vi "VI-Get KObject Descendants.vi"(11 "error in (no error)":errorcluster) -> (4 "KObject descendants":string[](array[string]), 15 "error out":errorcluster)   [LabVIEW 2015]
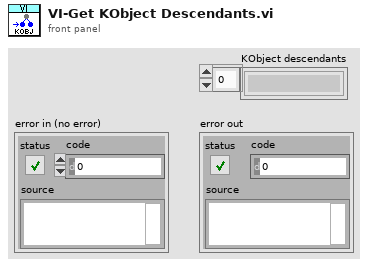
[diagram p1: front panel]
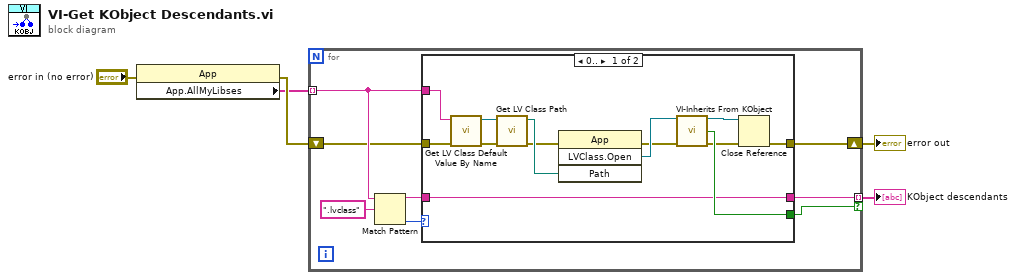
[diagram p0: block diagram]
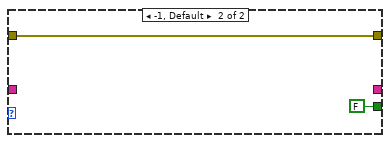
[diagram p2: hidden frame]
diagram:
  n1 = property class="App"(error in="error in (no error)") -> (error out=w3:errorcluster, "App.AllMyLibses"=w2:string[])  [unwired: 1 in, 1 out]
  n2 = for {
    tunnel: w2 -> [w11] mode=indexing
    shift-right: [w9] -> w4
    shift-left: w3 -> [w10]
    tunnel: [w7] -> w1 mode=indexing if=w6
    n3 = Match Pattern(string=w11, regular expression=".lvclass") -> (before substring=w8:string, offset past match=w12:i32)  [unwired: 1 in, 2 out]
    n4 = case shown="0.." w12 {
      tunnel: w11 -> [w23 _]
      tunnel: [w21 FALSE ("inherits?")] -> w6
      tunnel: w10 -> [w18 w28]
      tunnel: [w15 w28] -> w9
      tunnel: w8 -> [w14 _]
      tunnel: [w14 _] -> w7
      frame 0.. {
        n5 = call <vilib>:"Get LV Class Default Value By Name.vi"("error in (no error)"=w18, "class name"=w23) -> ("error out"=w26:errorcluster, "object"=w25:refnum<class>)  [unwired: 8 in]
        n6 = call <vilib>:"Get LV Class Path.vi"("error in (no error)"=w26, "object"=w25) -> ("error out"=w17:errorcluster, "class path"=w24:path)  [unwired: 8 in]
        n7 = invoke class="App" method="LVClass.Open"(error in=w17, "Path"=w24) -> (error out=w16:errorcluster, "LVClass.Open"=w22:refnum<vi>)  [unwired: 2 in, 2 out]
        n8 = call "VI-Inherits From KObject.vi"("LVClass Ref"=w22, "error in (no error)"=w16) -> ("LVClass Ref out"=w19:refnum<vi>, "inherits?"=w21:bool, "error out"=w20:errorcluster)  [unwired: 11 in]
        n9 = Close Reference(reference=w19, error in (no error)=w20) -> (error out=w15:errorcluster)
      }
      frame -1, Default {
      }
    }
  }
  "error out" <- w4
  "KObject descendants" <- w1
